vi "CalculateMcsaSpeed.vi"(6 "Calculation Cache In":T3 {"speed initial conditions"."zoom FFT settings"."FFT settings"."window" items=["Rectangle"=0, "Hanning"=1, "Hamming"=2, "Blackman-Harris"=3, "Exact Blackman"=4, "Blackman"=5, "Flat Top"=6, "4 Term B-Harris "=7, "7 Term B-Harris"=8, "Low Sidelobe"=9, "Blackman Nuttall"=11, "Triangle"=30, "Bartlett-Hanning"=31, "Bohman"=32, "Parzen"=33, "Welch"=34, "Kaiser"=60, "Dolph-Chebyshev"=61, "Gaussian"=62]; "spectrum initial conditions"."zoom FFT settings"."FFT settings"."window" items=["Rectangle"=0, "Hanning"=1, "Hamming"=2, "Blackman-Harris"=3, "Exact Blackman"=4, "Blackman"=5, "Flat Top"=6, "4 Term B-Harris "=7, "7 Term B-Harris"=8, "Low Sidelobe"=9, "Blackman Nuttall"=11, "Triangle"=30, "Bartlett-Hanning"=31, "Bohman"=32, "Parzen"=33, "Welch"=34, "Kaiser"=60, "Dolph-Chebyshev"=61, "Gaussian"=62]}, 7 "nameplate information":T2, 8 "error in (no error)":errorcluster, 9 "Map":T1, 10 "current waveform":waveform(dbl)[](array[waveform]), 11 "voltage waveform":waveform(dbl)[](array[waveform])) -> (0 "error out":errorcluster, 3 "speed [RPM]":dbl, 4 "Calculation Cache Out":T3 {"speed initial conditions"."zoom FFT settings"."FFT settings"."window" items=["Rectangle"=0, "Hanning"=1, "Hamming"=2, "Blackman-Harris"=3, "Exact Blackman"=4, "Blackman"=5, "Flat Top"=6, "4 Term B-Harris "=7, "7 Term B-Harris"=8, "Low Sidelobe"=9, "Blackman Nuttall"=11, "Triangle"=30, "Bartlett-Hanning"=31, "Bohman"=32, "Parzen"=33, "Welch"=34, "Kaiser"=60, "Dolph-Chebyshev"=61, "Gaussian"=62]; "spectrum initial conditions"."zoom FFT settings"."FFT settings"."window" items=["Rectangle"=0, "Hanning"=1, "Hamming"=2, "Blackman-Harris"=3, "Exact Blackman"=4, "Blackman"=5, "Flat Top"=6, "4 Term B-Harris "=7, "7 Term B-Harris"=8, "Low Sidelobe"=9, "Blackman Nuttall"=11, "Triangle"=30, "Bartlett-Hanning"=31, "Bohman"=32, "Parzen"=33, "Welch"=34, "Kaiser"=60, "Dolph-Chebyshev"=61, "Gaussian"=62]})   [LabVIEW 2017, in "McsaAnalysisFunctions.lvlib"]
uses:
  <vilib>/addons/InsightCM/Utilities/Analysis/MCSA/McsaAnalysisFunctions.lvlib
  <vilib>/addons/InsightCM/Utilities/Analysis/MCSA/controls/McsaCalculationCache.ctl
  <vilib>/addons/Electrical Power/Motor Monitoring/subVIs/ep_Initial Conditions for MCSA Spectra.ctl
  <vilib>/addons/Electrical Power/Motor Monitoring/subVIs/ep_Demodulation Algorithm.ctl
  <vilib>/addons/Electrical Power/Motor Monitoring/subVIs/ep_Zoom FFT Settings.ctl
  <vilib>/addons/Electrical Power/Motor Monitoring/subVIs/ep_Initial Conditions for Speed Estimation.ctl
  <vilib>/addons/PointValueMap/controls/PointMap.ctl
  <vilib>/addons/Electrical Power/Motor Monitoring/Speed Estimation (1 Motor with IC).vi
  <vilib>/addons/Electrical Power/Motor Monitoring/NI_EP_Motor Monitoring.lvlib
  <vilib>/addons/PointValueMap/PointValueMap.lvlib
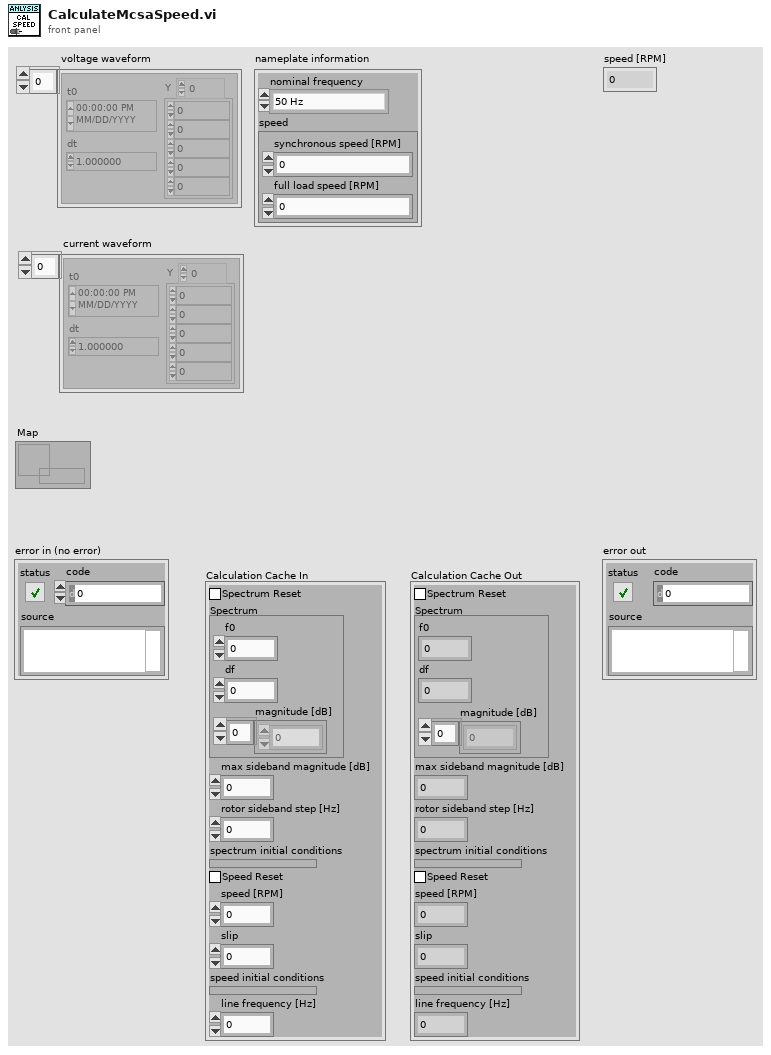
[diagram p1: front panel]
types:
  T1 = typedef "PointValueMap.lvlib/PointMap.ctl" = refnum<data-value>
  T2 = cluster{"nominal frequency":enum16{"50 Hz", "60 Hz"}, "speed":cluster{"synchronous speed [RPM]":dbl, "full load speed [RPM]":dbl}}
  T3 = typedef "McsaAnalysisFunctions.lvlib/McsaCalculationCache.ctl" = cluster{"Spectrum Reset":bool, "Spectrum":cluster{"f0":dbl, "df":dbl, "magnitude [dB]":dbl[]}, "max sideband magnitude [dB]":dbl, "rotor sideband step [Hz]":dbl, "spectrum initial conditions":T4, "Speed Reset":bool, "speed [RPM]":dbl, "slip":dbl, "speed initial conditions":T7, "line frequency [Hz]":dbl}
  T4 = typedef "NI_EP_Motor Monitoring.lvlib/ep_Initial Conditions for MCSA Spectra.ctl" = cluster{"hilbert state":cluster{"delay conditions":dbl[], "filter conditions":dbl[]}, "zoom FFT state":cluster{"phase state":dbl, "zoom FFT state":cluster{"zoom settings state":cluster{"zoom":i32, "stop band attenuation":enum16{"84 dB", "96 dB", "120 dB"}, "alias protect in final transition":bool, "oversampling ratio":dbl}, "SML Decimation Filter (complex input) state":cluster{"decimation settings state":cluster{"M":i32, "stop band attenuation":enum16{"84 dB", "96 dB", "120 dB"}, "alias protect in transition band":bool, "oversampling ratio":dbl}, "counter for garbage samples state":i32, "sml_Parameter Setting for Zoom Factor state":cluster{"filter length * interpolation state":i32, "interpolation state":i32, "comb filter order state":i32, "CFIR par state":cluster{"h":dbl[], "M":i32, "N":i32}, "LFIR par state":cluster{"h":dbl[], "M":i32, "N":i32}, "CIC Stages state":i32}, "aal_CIC (complex input) state":cluster{"aal_cascaded moving average (complex input) state":cluster{"states":cdb[], "circular buffers state":cdb[][], "circular buffer counter state":i32}, "aal_moving average with decimation by order (complex input) state":cluster{"residue result state":cdb, "processed data counter state":i32}}, "sml_Cascaded Decimation Filter (complex input) CFIR state":cluster{"unprocessed data state":cdb[], "final conditions state":cdb[][], "sml_M-1 Decimator with IC (complex input) state":cluster{"coefficients in reverse order state":dbl[], "max index for coefficients state":i32}}, "sml_Cascaded Decimation Filter (complex input) LFIR state":cluster{"unprocessed data state":cdb[], "final conditions state":cdb[][], "sml_M-1 Decimator with IC (complex input) state":cluster{"coefficients in reverse order state":dbl[], "max index for coefficients state":i32}}}, "ma_SML Data Packing (complex input) state":cluster{"array getting packed state":cdb[], "last array processed state":cdb[], "index state":i32, "packing parameters state":cluster{i32, "size":i32}}}, "FFT{X} [Vrms]":cdb[]}, "IIR filter state":cluster{"filter state":dbl[]}, "demodulation settings":cluster{"enable? (F)":bool, "algorithm":T5}, "highpass IIR Filter":cluster{"filter structure":enum32{"IIR 2nd Order", "IIR 4th Order"}, "Reverse Coefficients":dbl[], "Forward Coefficients":dbl[]}, "Hilbert FIR filter":cluster{"coefficients":dbl[], "delay":i32}, "zoom FFT settings":T6}
  T5 = typedef "NI_EP_Motor Monitoring.lvlib/ep_Demodulation Algorithm.ctl" = enum16{"1-phase signal", "3-phase signals"}
  T6 = typedef "NI_EP_Motor Monitoring.lvlib/ep_Zoom FFT Settings.ctl" = cluster{"FFT settings":cluster{"window":u16, "Window Size":i32, "FFT Size":i32, "%overlap":dbl}, "zoom settings":cluster{"zoom":i32, "stop band attenuation":enum16{"84 dB", "96 dB", "120 dB"}, "alias protect in final transition":bool, "oversampling ratio":dbl}, "other settings":cluster{"fmod":dbl, "f0":dbl, "df":dbl, "oidx":i32, "olen":i32}, "iterations":i32, "max block size":i32, "fs":dbl}
  T7 = typedef "NI_EP_Motor Monitoring.lvlib/ep_Initial Conditions for Speed Estimation.ctl" = cluster{"SVAF state":cluster{"space vector amplitude":dbl, "hilbert state":cluster{"delay conditions":dbl[], "filter conditions":dbl[]}}, "zoom FFT state":cluster{"phase state":dbl, "zoom FFT state":cluster{"zoom settings state":cluster{"zoom":i32, "stop band attenuation":enum16{"84 dB", "96 dB", "120 dB"}, "alias protect in final transition":bool, "oversampling ratio":dbl}, "SML Decimation Filter (complex input) state":cluster{"decimation settings state":cluster{"M":i32, "stop band attenuation":enum16{"84 dB", "96 dB", "120 dB"}, "alias protect in transition band":bool, "oversampling ratio":dbl}, "counter for garbage samples state":i32, "sml_Parameter Setting for Zoom Factor state":cluster{"filter length * interpolation state":i32, "interpolation state":i32, "comb filter order state":i32, "CFIR par state":cluster{"h":dbl[], "M":i32, "N":i32}, "LFIR par state":cluster{"h":dbl[], "M":i32, "N":i32}, "CIC Stages state":i32}, "aal_CIC (complex input) state":cluster{"aal_cascaded moving average (complex input) state":cluster{"states":cdb[], "circular buffers state":cdb[][], "circular buffer counter state":i32}, "aal_moving average with decimation by order (complex input) state":cluster{"residue result state":cdb, "processed data counter state":i32}}, "sml_Cascaded Decimation Filter (complex input) CFIR state":cluster{"unprocessed data state":cdb[], "final conditions state":cdb[][], "sml_M-1 Decimator with IC (complex input) state":cluster{"coefficients in reverse order state":dbl[], "max index for coefficients state":i32}}, "sml_Cascaded Decimation Filter (complex input) LFIR state":cluster{"unprocessed data state":cdb[], "final conditions state":cdb[][], "sml_M-1 Decimator with IC (complex input) state":cluster{"coefficients in reverse order state":dbl[], "max index for coefficients state":i32}}}, "ma_SML Data Packing (complex input) state":cluster{"array getting packed state":cdb[], "last array processed state":cdb[], "index state":i32, "packing parameters state":cluster{i32, "size":i32}}}, "FFT{X} [Vrms]":cdb[]}, "speed state":cluster{"speed [RPM]":dbl, "slip":dbl}, "speed estimation settings":cluster{"% overlap":dbl, "algorithm":T5}, "filter information":cluster{"coefficients":dbl[], "order":i32}, "zoom FFT settings":T6, "last valid window":i32, "fund. frequency for averager":dbl[]}
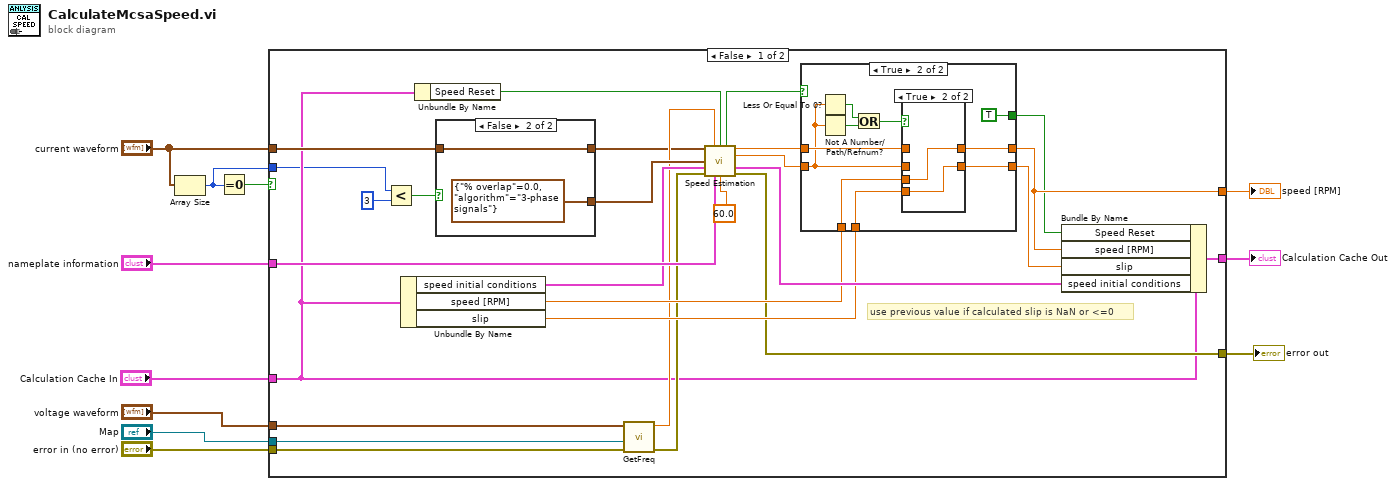
[diagram p0: block diagram]
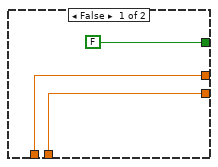
[diagram p2: hidden frame]
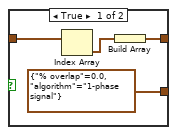
[diagram p4: hidden frame]
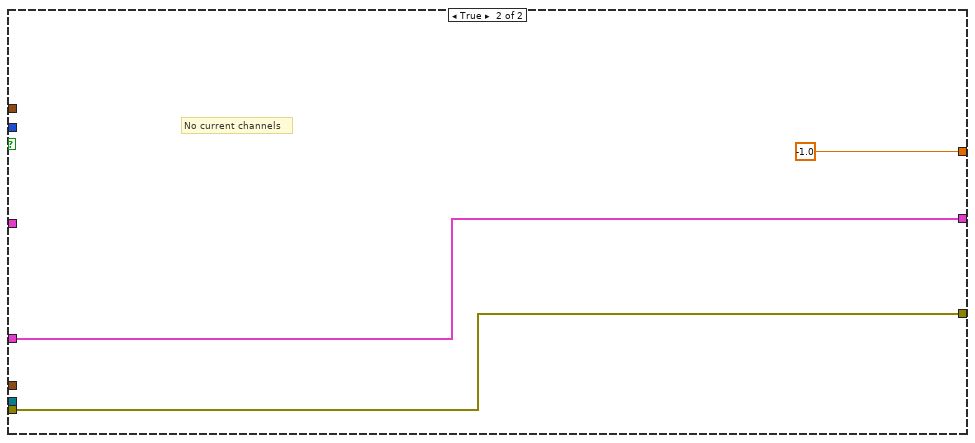
[diagram p5: hidden frame]
diagram:
  n1 = Array Size(array="current waveform") -> (size(s)=w1:i32)
  n2 = Equal To 0?(x=w1) -> (x = 0?=w2:bool)
  n3 = case shown="False" w2 {
    tunnel: "current waveform" -> [w38 _]
    tunnel: [w37 w63] -> w11
    tunnel: [w36 -1.0 ("speed [RPM]")] -> w10
    tunnel: "nameplate information" -> [w35 _]
    tunnel: [w18 w62] -> w8
    tunnel: "error in (no error)" -> [w17 w62]
    tunnel: "Calculation Cache In" -> [w16 w63]
    tunnel: "Map" -> [w15 _]
    tunnel: "voltage waveform" -> [w14 _]
    tunnel: w1 -> [w13 _]
    frame False {
      # "use previous value if calculated slip is NaN or <=0"
      n4 = Less?(x=w13, y=3) -> (x < y?=w33:bool)
      n5 = Unbundle By Name(w16) -> ("speed initial conditions"=w30:T7, "speed [RPM]"=w22:dbl, "slip"=w21:dbl)
      n6 = Unbundle By Name(w16) -> ("Speed Reset"=w32:bool)
      n7 = case shown="False" w33 {
        tunnel: w38 -> [w59 w61]
        tunnel: [w57 w61] -> w12
        tunnel: [cluster{"% overlap":dbl, "algorithm":T5} {"% overlap"=0.0, "algorithm"=enum."1-phase signal"} ("speed estimation settings") cluster{"% overlap":dbl, "algorithm":T5} {"% overlap"=0.0, "algorithm"=enum."3-phase signals"} ("speed estimation settings")] -> w31
        frame True {
          n8 = Index Array(array=w59) -> (element=w58:waveform(dbl))  [unwired: 1 in]
          n9 = Build Array(w58) -> (w57:waveform(dbl)[])
        }
        frame False {
        }
      }
      n10 = call <vilib>:"GetFreq.vi"("error in (no error)"=w17, "Map"=w15, "waveforms"=w14) -> ("error out"=w19:errorcluster, "frequency"=w20:dbl)  [unwired: 7 in]
      n11 = call-poly <vilib>:"Speed Estimation.vi"("waveforms"=w12, "fundamental frequency [Hz]"=w20, "reset? (F)"=w32, "speed estimation settings"=w31, "initial conditions"=w30, "error in (no error)"=w19, "nameplate information"=w35, "window length (60 s)"=60.0) -> ("new data available?"=w26:bool, "speed [RPM]"=w25:dbl, "slip"=w23:dbl, "final conditions"=w28:T7, "error out"=w18:errorcluster)  [unwired: 3 in]
      n12 = case shown="True" w26 {
        tunnel: [FALSE ("Speed Reset") TRUE ("Speed Reset")] -> w27
        tunnel: [w40 w45] -> w36
        tunnel: w25 -> [_ w47]
        tunnel: [w39 w44] -> w24
        tunnel: w23 -> [_ w46]
        tunnel: w22 -> [w40 w43]
        tunnel: w21 -> [w39 w42]
        frame False {
        }
        frame True {
          n13 = Less Or Equal To 0?(x=w46) -> (x <= 0?=w50:bool)
          n14 = Not A Number/Path/Refnum?(number/path/refnum=w46) -> (NaN/Path/Refnum?=w49:bool)
          n15 = Or(x=w50, y=w49) -> (x .or. y?=w48:bool)
          n16 = case shown="True" w48 {
            tunnel: w47 -> [w53 _]
            tunnel: w46 -> [w52 _]
            tunnel: [w53 w55] -> w45
            tunnel: [w52 w54] -> w44
            tunnel: w43 -> [_ w55]
            tunnel: w42 -> [_ w54]
            frame False {
            }
            frame True {
            }
          }
        }
      }
      n17 = Bundle By Name(cluster=w16, "Speed Reset"=w27, "speed [RPM]"=w36, "slip"=w24, "speed initial conditions"=w28) -> (w37:T3)
    }
    frame True {
      # "No current channels"
    }
  }
  "speed [RPM]" <- w10
  "Calculation Cache Out" <- w11
  "error out" <- w8
